vi "GetPSUStatus.vi"(8 "error in (no error)":errorcluster, 11 "PSU in":refnum<class "PSU.lvclass">) -> (0 "error out":errorcluster, 1 "OCP Tripped":bool, 2 "OVP Tripped":bool, 3 "PSU out":refnum<class "PSU.lvclass">, 4 "Current (A)":dbl, 5 "Voltage (V)":dbl)   [LabVIEW 2014, in "PSU.lvclass"]
uses:
  PSU.lvclass
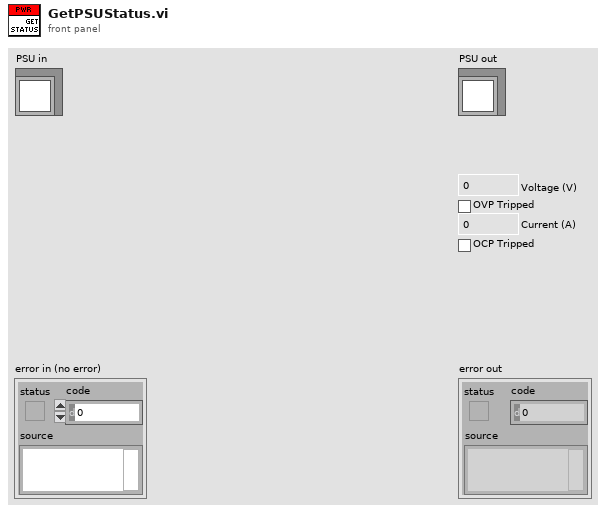
[diagram p1: front panel]
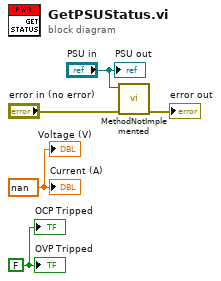
[diagram p0: block diagram]
diagram:
  w1 = FALSE
  w2 = nan ("Current (A)")
  n1 = call "MethodNotImplemented.vi"("error in (no error)"="error in (no error)", "LabVIEW Object In"="PSU in") -> ("error out"=→"error out":errorcluster)  [unwired: 9 in]
  "PSU out" <- "PSU in"
  "Voltage (V)" <- w2
  "Current (A)" <- w2
  "OCP Tripped" <- w1
  "OVP Tripped" <- w1
